vi "Int_Status_String_Status.vi"(1 "[STATUS]":i32) -> (0 "STATUS":string)   [LabVIEW 2020]
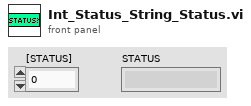
[diagram p1: front panel]
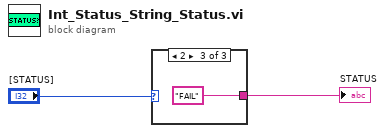
[diagram p0: block diagram]
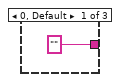
[diagram p2: hidden frame]
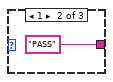
[diagram p3: hidden frame]
diagram:
  n1 = case shown="2" "[STATUS]" {
    tunnel: ["" ("[DTS_PASS]") "PASS" ("[DTS_PASS]") "FAIL" ("[DTS_PASS]")] -> w2
    frame 0, Default {
    }
    frame 1 {
    }
    frame 2 {
    }
  }
  "STATUS" <- w2
